vi "test_DeviceManager_OpenWebSocketCommunication.vi"(8 "error in":errorcluster) -> (0 "error out":errorcluster)   [LabVIEW 2023, in "horiba.test.lvlib"]
doc: "_____\nCreated using DQMH Event Scripter 7.0.0.1280."
uses:
  <vilib>/addons/_JKI Toolkits/Caraya/classes/Assert/Assert Not Error.vi
  <vilib>/addons/_JKI Toolkits/Caraya/classes/Assert/Assert True.vi
  horiba.test.lvlib
  Classes/DeviceManager/DeviceManager.lvlib
  <vilib>/addons/_JKI Toolkits/Caraya/classes/Test/Test.lvclass
  <vilib>/addons/_JKI Toolkits/Caraya/classes/Assert/Assert.lvclass
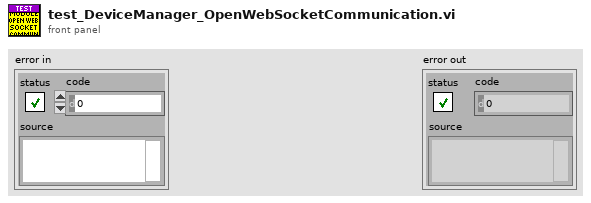
[diagram p1: front panel]
types:
  T1 = typedef "horiba.lvlib/DeviceManager.lvlib/Broadcast Events--cluster.ctl" = cluster{"Module Did Init":refnum<user-event>, "Status Updated":refnum<user-event>, "Error Reported":refnum<user-event>, "Module Did Stop":refnum<user-event>, "Update Module Execution Status":refnum<user-event>, "iclIsRunning":refnum<user-event>, "websocketConnectionOpened":refnum<user-event>, "devicesDiscovered":refnum<user-event>}
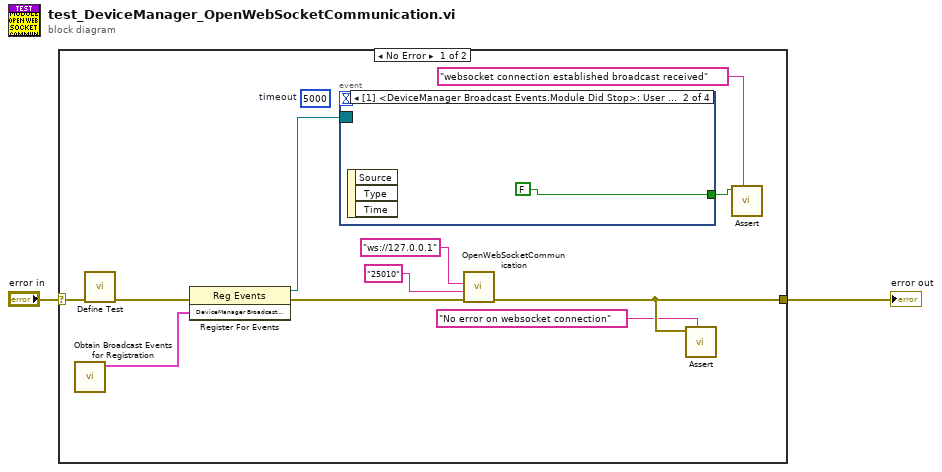
[diagram p0: block diagram]
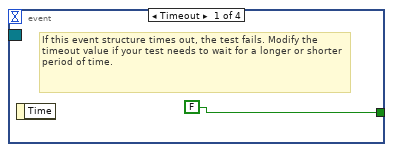
[diagram p2: hidden frame]
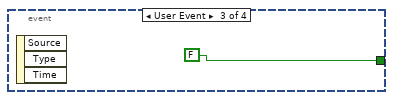
[diagram p3: hidden frame]
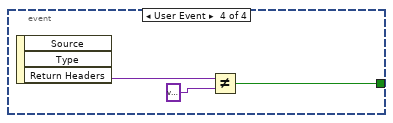
[diagram p4: hidden frame]
diagram:
  n1 = case shown="No Error" "error in" {
    selector: "error in" -> [w13 w20]
    tunnel: [w4 w20] -> w1
    frame No Error {
      (unwired) 5000  # timeout
      n2 = call "Obtain Broadcast Events for Registration.vi"() -> ("DeviceManager Broadcast Events"=w10:T1)  [unwired: 9 in, 2 out]
      n3 = call <vilib>:"Define Test.vi"("error in (no error)"=w13) -> ("error out"=w8:errorcluster)  [unwired: 9 in, 1 out]
      n4 = register-events(error in=w8, w10) -> (reference out=w6:refnum<event-registration>, error out=w7:errorcluster)  [unwired: 1 in]
      n5 = event shown="[1] <DeviceManager Broadcast Events.Module Did Stop>: User Event" {
        selector: w6 -> [_ _ _ _]
        dyn-events: _ -> [_ _ _ _]
        timeout: _ -> [_ _ _ _]
        tunnel: [FALSE FALSE FALSE w17] -> w5
        event Timeout {
          # "If this event structure times out, the test fails. Modify the timeout value if your test needs to wait for a longer or shorter period of time."
          n6 = event-data() -> ()  [unwired: 1 in, 1 out]
        }
        event User Event {
          n7 = event-data() -> ()  [unwired: 1 in, 3 out]
        }
        event User Event {
          n8 = event-data() -> ()  [unwired: 1 in, 3 out]
        }
        event User Event {
          n9 = event-data() -> ("Return Headers"=w19:variant)  [unwired: 1 in, 2 out]
          n10 = Not Equal?(x=w19, y=variant) -> (x != y?=w17:bool)
        }
      }
      n11 = call "OpenWebSocketCommunication.vi"("error in"=w7, "WS Server Port"="25010", "WS Server IP"="ws://127.0.0.1") -> ("error out"=w4:errorcluster)  [unwired: 6 in, 2 out]
      n12 = call-poly <vilib>:"Assert.vi"("Label"="No error on websocket connection", "Not Error?"=w4) -> ()  [unwired: 8 in, 2 out]
      n13 = call-poly <vilib>:"Assert.vi"("Label"="websocket connection established broadcast received", "True?"=w5) -> ()  [unwired: 8 in, 2 out]
    }
    frame Error {
    }
  }
  "error out" <- w1
